vi "Lot_Unload.vi"(8 "error in (no error)":errorcluster, 11 "LotData in":refnum<class "LotData.lvclass">) -> (0 "error out":errorcluster, 3 "LotData out":refnum<class "LotData.lvclass">)   [LabVIEW 2012, in "LotData.lvclass"]
uses:
  LotData.lvclass
  Controls/TestData.ctl
  Controls/WaferTable.ctl
  Controls/LotData_Current.ctl
  LotData.lvclass/LotData.ctl
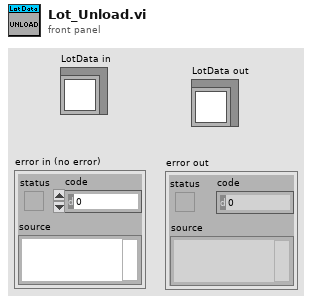
[diagram p1: front panel]
types:
  T1 = cluster{"Area":string, "Wavelength":dbl[], "EL Spectrum":dbl[]}
  T2 = typedef "TestData.ctl" = cluster{"20mA Data":cluster{"Area":string, "Current,mA":dbl, "Power":dbl, "WL":dbl, "Voltage":dbl, "Knee Current":dbl, "Reverse":dbl}, "50mA Data":cluster{"Area":string, "Current,mA":dbl, "Power":dbl, "WL":dbl, "Voltage":dbl}}
  T3 = typedef "LotData.lvclass/LotData_Current.ctl" = cluster{"area":i32, "Data":cluster{"wl":dbl, "power":dbl, "voltage":dbl, "knee":dbl, "reverse":dbl}}
  T4 = typedef "WaferTable.ctl" = string[][]
  T5 = cluster{"Area":string, "Current,mA":dbl, "Power":dbl, "WL":dbl, "Voltage":dbl, "Knee Current":dbl, "Reverse":dbl}
  T6 = cluster{"Area":string, "Current,mA":dbl, "Power":dbl, "WL":dbl, "Voltage":dbl}
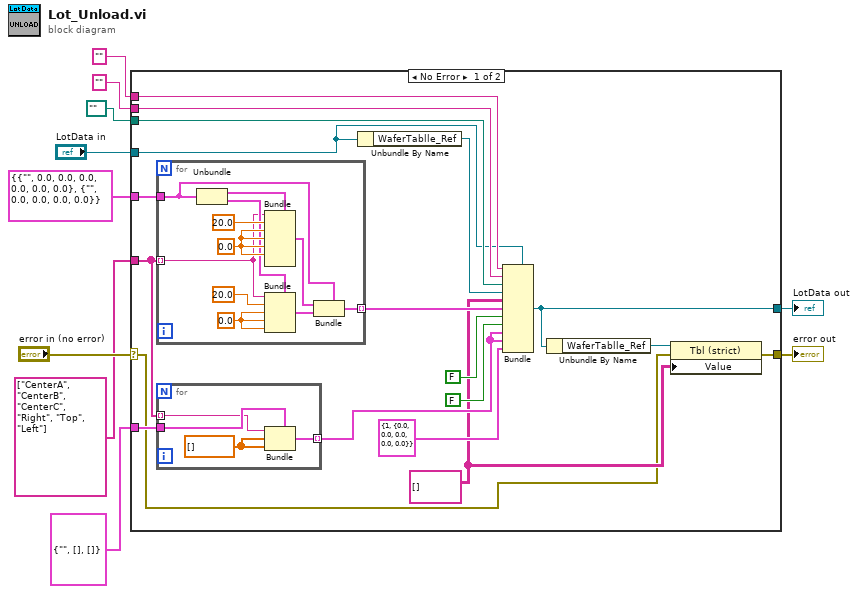
[diagram p0: block diagram]
diagram:
  n1 = case shown="No Error" "error in (no error)" {
    selector: "error in (no error)" -> [w13 w45]
    tunnel: [w11 w45] -> w9
    tunnel: [w12 w44] -> w7
    tunnel: "LotData in" -> [w16 w44]
    tunnel: "" ("Wafer ID") -> [w24 _]
    tunnel: "" ("Type") -> [w23 _]
    tunnel: path "" ("FilePath") -> [w22 _]
    tunnel: T2 {"20mA Data"={"Area"="", "Current,mA"=0.0, "Power"=0.0, "WL"=0.0, "Voltage"=0.0, "Knee Current"=0.0, "Reverse"=0.0}, "50mA Data"={"Area"="", "Current,mA"=0.0, "Power"=0.0, "WL"=0.0, "Voltage"=0.0}} ("TestData") -> [w21 _]
    tunnel: string[] ["CenterA", "CenterB", "CenterC", "Right", "Top", "Left"] -> [w20 _]
    tunnel: T1 {"Area"="", "Wavelength"=[], "EL Spectrum"=[]} ("Spect") -> [w19 _]
    frame No Error {
      w14 = T4 [] ("WaferTable")
      n2 = for {
        tunnel: w21 -> [w36]
        tunnel: w20 -> [w37] mode=indexing
        tunnel: [w33] -> w28 mode=indexing
        w40 = 0.0 ("Power")
        w41 = 0.0 ("Power")
        n3 = Unbundle(w36) -> ("20mA Data"=w43:T5, "50mA Data"=w38:T6)
        n4 = Bundle(cluster=w43, "Area"=w37, "Current,mA"=20.0, "Power"=w41, "WL"=w41, "Voltage"=w41, "Knee Current"=w41) -> (w35:T5)  [unwired: 1 in]
        n5 = Bundle(cluster=w38, "Area"=w37, "Current,mA"=20.0, "Power"=w40, "WL"=w40, "Voltage"=w40) -> (w34:T6)
        n6 = Bundle(cluster=w36, "20mA Data"=w35, "50mA Data"=w34) -> (w33:T2)
      }
      n7 = for {
        tunnel: w20 -> [w31] mode=indexing
        tunnel: w19 -> [w32]
        tunnel: [w29] -> w25 mode=indexing
        w30 = dbl[] [] ("Wavelength")
        n8 = Bundle(cluster=w32, "Area"=w31, "Wavelength"=w30, "EL Spectrum"=w30) -> (w29:T1)
      }
      n9 = Unbundle By Name(w16) -> ("WaferTablle_Ref"=w17:refnum<vi>)
      n10 = Bundle(cluster=w16, w24, w23, w22, w17, w14, w28, FALSE ("Loaded"), FALSE ("Saved"), w25, w25, T3 {"area"=1, "Data"={"wl"=0.0, "power"=0.0, "voltage"=0.0, "knee"=0.0, "reverse"=0.0}} ("Current")) -> (w12:refnum<class "LotData.lvclass">)
      n11 = Unbundle By Name(w12) -> ("WaferTablle_Ref"=w15:refnum<vi>)
      n12 = property class="Tbl (strict)"(reference=w15, error in=w13, "Value"=w14) -> (error out=w11:errorcluster)  [unwired: 1 out]
    }
    frame Error {
    }
  }
  "error out" <- w9
  "LotData out" <- w7
